vi "ECG BY DAQ.vi"() -> ()   [LabVIEW 2024]
uses:
  <vilib>/addons/Biomedical/Biosignal Measurements/ECG/subVIs/ECG features.ctl
  <vilib>/addons/Biomedical/NI_BMTK_Measurements.lvlib
panel:
  out "PR Segment Not in Range":bool
  out "PR Segmant In RAnge":bool
  out "P Wave In Range":bool
  out "P Wave Not in Range":bool
  out "PR interval Not in Range":bool
  out "PR interval In  Range":bool
  out "QRS Complex in Range":bool
  out "QT interval in Range":bool
  out "QT interval not in Range":bool
  out "T Wave Not in Range":bool
  out "QRS Complex Not in Range":bool
  out "ST Segment in Range":bool
  out "T Wave in Range":bool
  out "ST Segment Not in Range":bool
  in  "stop (F)":bool
  out "Statistics":T1
  out "Array of Features":T2[](array[typedef])
  out "Number of peaks":i32
  out "Location":dbl[](array[numeric])
  out "Amplitude":dbl[](array[numeric])
  out "Peak plot":cluster{"Ramp Pattern":dbl[], "X":dbl[]}[](graph)
  in  "peaks/valleys":u16(ring) items=["peaks", "valleys"]
  out "Tachycardia":bool
  out "Bradycardia":bool
  out "Normal":bool
  out "Heart Beat":dbl
  out "Number of cycles":i32
  out "Denoise Signal":waveform(dbl)(graph) caption="Denoised Signal"
  out "Raw Acquired Signal":dynamicdata(graph) caption="Raw Aquired Signal"
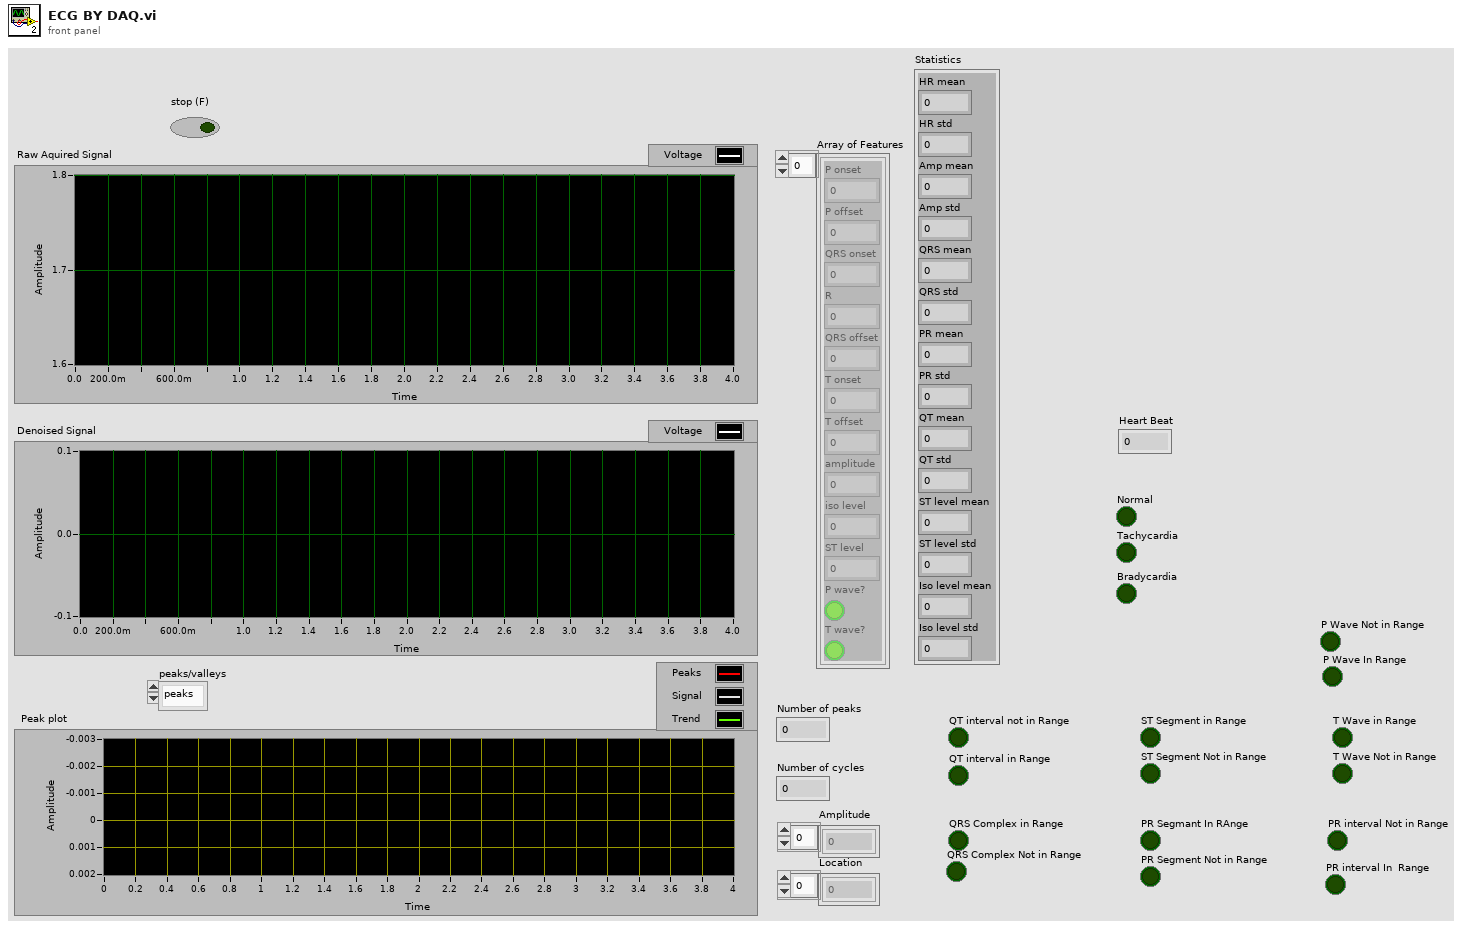
[diagram p1: front panel]
types:
  T1 = cluster{"HR mean":dbl, "HR std":dbl, "Amp mean":dbl, "Amp std":dbl, "QRS mean":dbl, "QRS std":dbl, "PR mean":dbl, "PR std":dbl, "QT mean":dbl, "QT std":dbl, "ST level mean":dbl, "ST level std":dbl, "Iso level mean":dbl, "Iso level std":dbl}
  T2 = typedef "NI_BMTK_Measurements.lvlib/ECG features.ctl" = cluster{"P onset":dbl, "P offset":dbl, "QRS onset":dbl, "R":dbl, "QRS offset":dbl, "T onset":dbl, "T offset":dbl, "amplitude":dbl, "iso level":dbl, "ST level":dbl, "P wave?":bool, "T wave?":bool}
  T3 = cluster{"detrend? (F)":bool, "threshold frequency":dbl}
  T4 = cluster{"Array of Features[0]":T2, "Array of Features[1]":T2, "Array of Features[2]":T2}
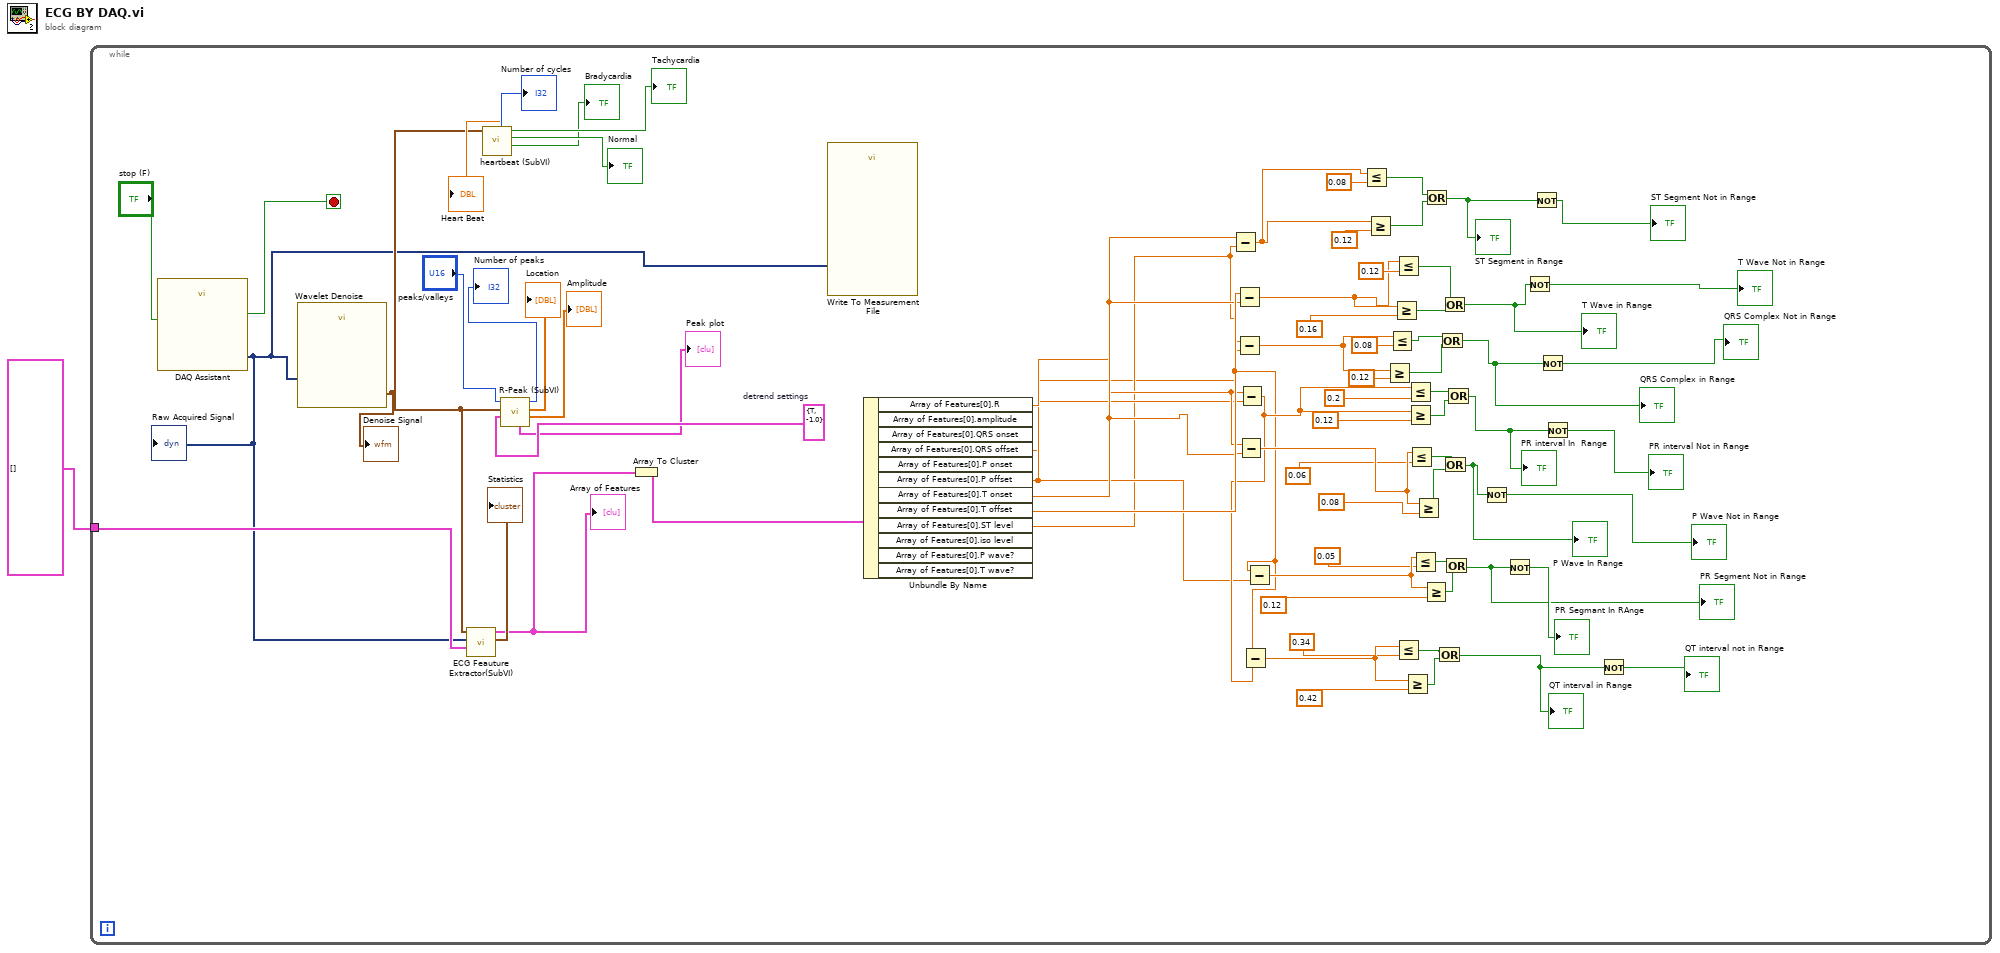
[diagram p0: block diagram]
diagram:
  n1 = while {
    tunnel: T2[] [] -> [w63]
    stop <- w58 stop-if-true
    w69 = T3 {"detrend? (F)"=TRUE, "threshold frequency"=-1.0}  # detrend settings
    n2 = call "DAQ Assistant"("stop (F)"="stop (F)") -> ("data"=w2:dynamicdata, "stopped"=w58:bool)  [unwired: 15 in, 2 out]
    "Raw Acquired Signal" <- w2
    n3 = call "Wavelet Denoise"("Signal"=w2) -> ("Denoised Signal"=w64:waveform(dbl))  [unwired: 9 in, 1 out]
    "Denoise Signal" <- w64
    n4 = call "ECG Feauture Extractor(SubVI).vi"("Array"=w63, "data"=w2, "Denoised Signal"=w64) -> ("Statistics"=→"Statistics":T1, "Array of Features"=w59:T2[])  [unwired: 7 in]
    "Array of Features" <- w59
    n5 = call "heartbeat (SubVI).vi"("Denoised Signal"=w64) -> ("Bradycardia"=→"Bradycardia":bool, "Normal"=→"Normal":bool, "Tachycardia"=→"Tachycardia":bool, "Number of cycles"=→"Number of cycles":i32, "Heart Rate"=→"Heart Beat":dbl)  [unwired: 6 in]
    n6 = call "R-Peak (SubVI).vi"("detrend settings"=w69, "Denoised Signal"=w64, "peaks/valleys"="peaks/valleys") -> ("Amplitude"=→"Amplitude":dbl[], "Location"=→"Location":dbl[], "Number of peaks"=→"Number of peaks":i32, "Peak plot"=→"Peak plot":cluster{"Ramp Pattern":dbl[], "X":dbl[]}[])  [unwired: 5 in]
    n7 = Array To Cluster(array=w59) -> (cluster=w60:T4)
    n8 = call "Write To Measurement File"("Signals"=w2) -> ()  [unwired: 16 in, 3 out]
    n9 = Unbundle By Name(w60) -> ("Array of Features[0].R"=w6:dbl, "Array of Features[0].QRS offset"=w3:dbl, "Array of Features[0].P offset"=w5:dbl, "Array of Features[0].T onset"=w8:dbl, "Array of Features[0].T offset"=w9:dbl, "Array of Features[0].ST level"=w4:dbl)  [unwired: 6 out]
    n10 = Subtract(x=w8, y=w4) -> (x-y=w27:dbl)
    n11 = Subtract(x=w9, y=w8) -> (x-y=w25:dbl)
    n12 = Subtract(x=w4, y=w3) -> (x-y=w23:dbl)
    n13 = Subtract(x=w6, y=w8) -> (x-y=w20:dbl)
    n14 = Subtract(x=w6, y=w5) -> (x-y=w7:dbl)
    n15 = Subtract(x=w3, y=w7) -> (x-y=w22:dbl)
    n16 = Subtract(x=w3, y=w5) -> (x-y=w21:dbl)
    n17 = Less Or Equal?(x=w27, y=0.08) -> (x <= y?=w31:bool)
    n18 = Greater Or Equal?(x=w27, y=0.12) -> (x >= y?=w30:bool)
    n19 = Greater Or Equal?(x=w23, y=0.12) -> (x >= y?=w35:bool)
    n20 = Less Or Equal?(x=w23, y=0.08) -> (x <= y?=w34:bool)
    n21 = Greater Or Equal?(x=w25, y=0.16) -> (x >= y?=w33:bool)
    n22 = Less Or Equal?(x=w25, y=0.12) -> (x <= y?=w32:bool)
    n23 = Less Or Equal?(x=w22, y=0.34) -> (x <= y?=w37:bool)
    n24 = Greater Or Equal?(x=w22, y=0.42) -> (x >= y?=w36:bool)
    n25 = Less Or Equal?(x=w7, y=0.2) -> (x <= y?=w42:bool)
    n26 = Greater Or Equal?(x=w7, y=0.12) -> (x >= y?=w43:bool)
    n27 = Less Or Equal?(x=w20, y=0.06) -> (x <= y?=w40:bool)
    n28 = Less Or Equal?(x=w21, y=0.05) -> (x <= y?=w39:bool)
    n29 = Greater Or Equal?(x=w20, y=0.08) -> (x >= y?=w41:bool)
    n30 = Greater Or Equal?(x=w21, y=0.12) -> (x >= y?=w38:bool)
    n31 = Or(x=w31, y=w30) -> (x .or. y?=w56:bool)
    "ST Segment in Range" <- w56
    n32 = Or(x=w37, y=w36) -> (x .or. y?=w45:bool)
    "QT interval in Range" <- w45
    n33 = Or(x=w34, y=w35) -> (x .or. y?=w52:bool)
    "QRS Complex in Range" <- w52
    n34 = Or(x=w32, y=w33) -> (x .or. y?=w54:bool)
    "T Wave in Range" <- w54
    n35 = Or(x=w40, y=w41) -> (x .or. y?=w48:bool)
    "P Wave In Range" <- w48
    n36 = Or(x=w39, y=w38) -> (x .or. y?=w46:bool)
    "PR Segment Not in Range" <- w46
    n37 = Or(x=w42, y=w43) -> (x .or. y?=w50:bool)
    "PR interval In  Range" <- w50
    n38 = Not(x=w48) -> (.not. x?=→"P Wave Not in Range":bool)
    n39 = Not(x=w46) -> (.not. x?=→"PR Segmant In RAnge":bool)
    n40 = Not(x=w54) -> (.not. x?=→"T Wave Not in Range":bool)
    n41 = Not(x=w56) -> (.not. x?=→"ST Segment Not in Range":bool)
    n42 = Not(x=w52) -> (.not. x?=→"QRS Complex Not in Range":bool)
    n43 = Not(x=w50) -> (.not. x?=→"PR interval Not in Range":bool)
    n44 = Not(x=w45) -> (.not. x?=→"QT interval not in Range":bool)
  }
